vi "Destroy.vi"(8 "error in (no error)":errorcluster, 11 "reference in":refnum<class "CompressionDecorator.lvclass">) -> (0 "error out":errorcluster, 3 "reference out":refnum<class "CompressionDecorator.lvclass">)   [LabVIEW 2020, in "CompressionDecorator.lvclass"]
uses:
  CompressionDecorator.lvclass
  DataSourceDecorator_class/DataSourceDecorator.lvclass
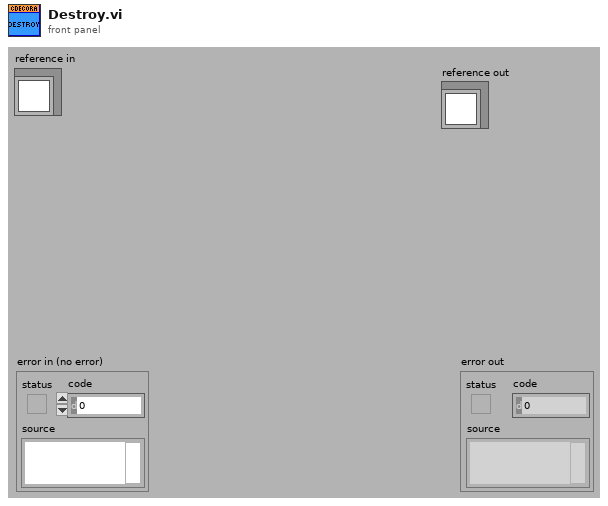
[diagram p1: front panel]
types:
  T1 = typedef "CompressionDecorator.lvclass/ObjectAttributes.ctl" = cluster{"CompLevel":i32}
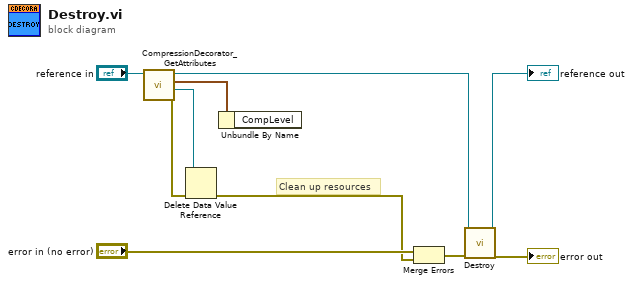
[diagram p0: block diagram]
diagram:
  # "Clean up resources"
  n1 = call "CompressionDecorator_GetAttributes.vi"("reference in"="reference in") -> ("error out"=w8:errorcluster, "DataRef"=w5:refnum<data-value>, "Data"=w7:T1, "reference out"=w6:refnum<class "CompressionDecorator.lvclass">)  [unwired: 7 in]
  n2 = Delete Data Value Reference(data value reference=w5, error in=w8) -> (error out=w3:errorcluster)  [unwired: 1 out]
  n3 = Unbundle By Name(w7) -> ()  [unwired: 1 out]
  n4 = Merge Errors("error in (no error)", w3) -> (w10:errorcluster)
  n5 = call-parent "Destroy.vi"("error in (no error)"=w10, "reference in"=w6) -> ("error out"=→"error out":errorcluster, "reference out"=→"reference out":refnum<class "CompressionDecorator.lvclass">)  [unwired: 8 in]
